vi "SavePath.vi"(10 "File Name":string=".csv", 11 "Path In":string="C:\\CS-BarCode\\Save Date\\") -> (3 "Folder Path":path, 5 "File Path":path)   [LabVIEW 2014]
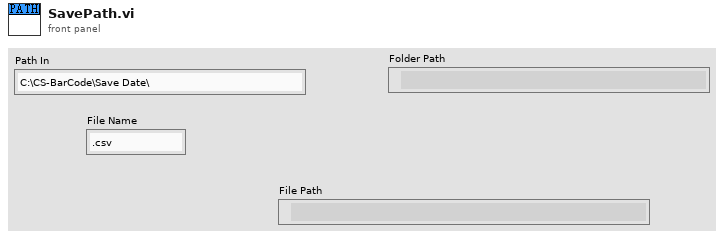
[diagram p1: front panel]
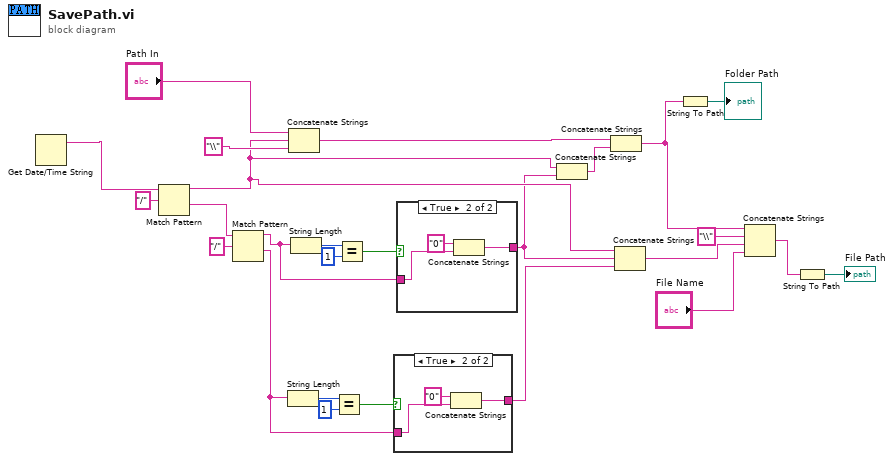
[diagram p0: block diagram]
diagram:
  n1 = Get Date/Time String() -> (date string=w26:string)  [unwired: 3 in, 1 out]
  n2 = Match Pattern(string=w26, regular expression="/") -> (before substring=w9:string, after substring=w22:string)  [unwired: 1 in, 2 out]
  n3 = Match Pattern(string=w22, regular expression="/") -> (before substring=w17:string, after substring=w11:string)  [unwired: 1 in, 2 out]
  n4 = String Length(string=w11) -> (length=w12:i32)
  n5 = Concatenate Strings("Path In", w9, "\\") -> (w16:string)
  n6 = String Length(string=w17) -> (length=w20:i32)
  n7 = Equal?(x=w12, y=1) -> (x = y?=w14:bool)
  n8 = Equal?(x=w20, y=1) -> (x = y?=w18:bool)
  n9 = case shown="True" w14 {
    tunnel: w11 -> [w27 w30]
    tunnel: [w27 w28] -> w7
    frame False {
    }
    frame True {
      n10 = Concatenate Strings("0" ("string"), w30) -> (w28:string)
    }
  }
  n11 = case shown="True" w18 {
    tunnel: w17 -> [w31 w34]
    tunnel: [w31 w32] -> w8
    frame False {
    }
    frame True {
      n12 = Concatenate Strings("0" ("string"), w34) -> (w32:string)
    }
  }
  n13 = Concatenate Strings(w9, w8) -> (w15:string)
  n14 = Concatenate Strings(w16, w15) -> (w4:string)
  n15 = Concatenate Strings(w9, w8, w7) -> (w6:string)
  n16 = String To Path(string=w4) -> (path=→"Folder Path":path)
  n17 = Concatenate Strings(w4, "\\" ("string"), w6, "File Name") -> (w2:string)
  n18 = String To Path(string=w2) -> (path=→"File Path":path)
